vi "CRYFlatten End.vi"() -> (3 "Flatten End String":string)   [LabVIEW 2013]
uses:
  Typedef Control/CRYEnd Cluster.ctl
panel:
  in  "End Cluster Step":T1
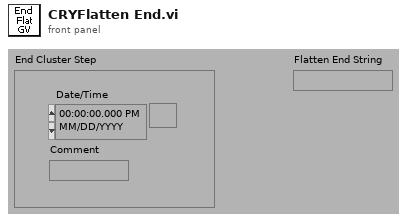
[diagram p1: front panel]
types:
  T1 = typedef "CRYEnd Cluster.ctl" = cluster{"Comment":string, "Date/Time":timestamp}
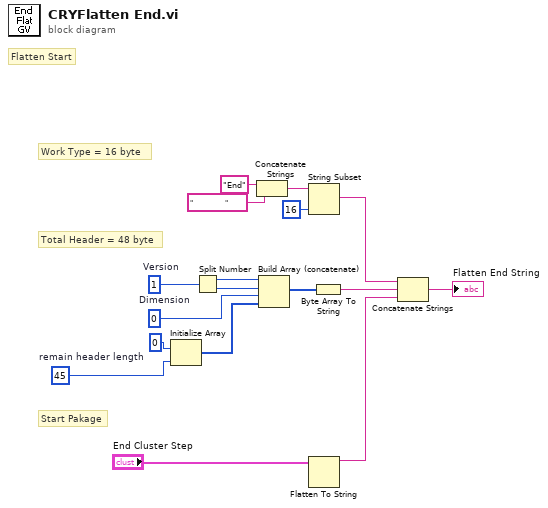
[diagram p0: block diagram]
diagram:
  w11 = u16 1  # Version
  w8 = u8 0  # Dimension
  w12 = 45  # remain header length
  # "Flatten Start"
  # "Start Pakage"
  # "Work Type = 16 byte"
  # "Total Header = 48 byte"
  n1 = Initialize Array(u8 0 ("element"), w12) -> (w6:u8[])
  n2 = Split Number(x=w11) -> (hi(x)=w10:u8, lo(x)=w9:u8)
  n3 = Concatenate Strings("End" ("string"), "                " ("string")) -> (w15:string)
  n4 = Build Array (concatenate)(w10, w9, w8, w6) -> (w7:u8[])
  n5 = String Subset(string=w15, length (rest)=16 ("length (rest)")) -> (substring=w2:string)  [unwired: 1 out]
  n6 = Flatten To String(anything="End Cluster Step") -> (data string=w5:string)  [unwired: 1 in, 4 out]
  n7 = Byte Array To String(unsigned byte array=w7) -> (string=w4:string)
  n8 = Concatenate Strings(w2, w4, w5) -> (→"Flatten End String":string)
